vi "Command Set.vi"   [LabVIEW 2018]
uses:
  Buttons.ctl
types:
  T1 = typedef "Buttons.ctl" = enum16{"A", "B", "X", "Y", "LB", "RB", "Back", "Start", "LS", "RS"}
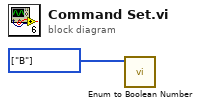
[diagram p0: block diagram]
diagram:
  w1 = T1[] [enum."B"] items=["A", "B", "X", "Y", "LB", "RB", "Back", "Start", "LS", "RS"] ("Button Selection")
  n1 = call "Enum to Boolean Number.vi"("Button Selection"=w1) -> ()  [unwired: 3 in, 1 out]
